vi "Avg Fuel String Append.vi"(1 "Append String":string=" 1h", 2 "Slave ID":dbl) -> (0 "Avg captions":string[](array[string]))   [LabVIEW 2017, in "GUI.lvlib"]
uses:
  GUI.lvlib
  Konfiguracja/Konfiguracja.lvlib
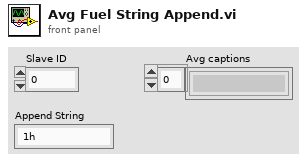
[diagram p1: front panel]
types:
  T1 = cluster{"Paliwo 1":string, "Paliwo 2":string, "Paliwo 3":string, "Paliwo 4":string, "Paliwo 5":string, "Paliwo 6":string}
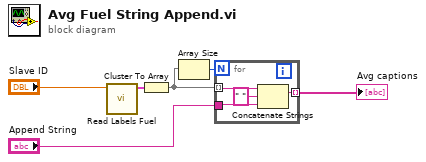
[diagram p0: block diagram]
diagram:
  n1 = call "Read Labels Fuel.vi"("Slave ID"="Slave ID") -> ("Etykiety P1-6"=w5:T1)  [unwired: 10 in]
  n2 = Cluster To Array(cluster=w5) -> (array=w2:string[])
  n3 = Array Size(array=w2) -> (size(s)=w1:i32)
  n4 = for {
    N: w1 -> [_]
    tunnel: w2 -> [w10] mode=indexing
    tunnel: [w9] -> w3 mode=indexing
    tunnel: "Append String" -> [w8]
    n5 = Concatenate Strings(w10, " " ("string"), w8) -> (w9:string)
  }
  "Avg captions" <- w3
